vi "Write Report.vi"(8 "error in (no error)":errorcluster, 10 "Resource In":variant, 11 "Analyze Compound Results Base in":refnum<class "Analyze Compound Results Base.lvclass">) -> (0 "error out":errorcluster, 2 "Resource Out":variant, 3 "Analyze Compound Results Base out":refnum<class "Analyze Compound Results Base.lvclass">)   [LabVIEW 2014, in "Analyze Compound Results Base.lvclass"]
uses:
  Analyze Compound Results Base.lvclass
  Analyze Compound Results Base.lvclass/Analyze Compound Results Base.ctl
  Results Base/Analyze Results Base.lvclass
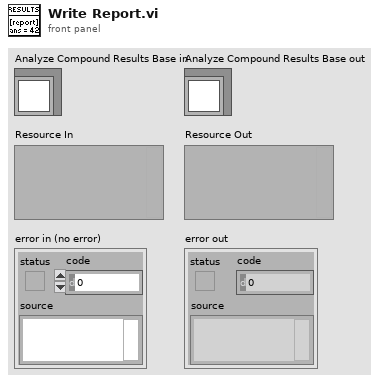
[diagram p1: front panel]
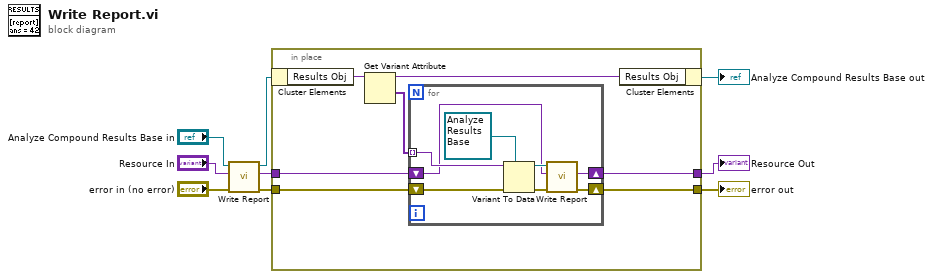
[diagram p0: block diagram]
diagram:
  n1 = call-parent "Write Report.vi"("error in (no error)"="error in (no error)", "Resource In"="Resource In", "Analyze Results Base in"="Analyze Compound Results Base in") -> ("error out"=w5:errorcluster, "Resource Out"=w2:variant, "Analyze Results Base out"=w6:refnum<class "Analyze Compound Results Base.lvclass">)  [unwired: 6 in]
  n2 = in-place {
    in-place-border: [w13] -> w4
    in-place-border: [w12] -> w3
    in-place-border: w5 -> [w11]
    in-place-border: w2 -> [w10]
    n3 = in-place-cluster #1(w6) -> ("Results Obj"=w16:variant)
    n4 = Get Variant Attribute(Variant=w16) -> (duplicate Variant=w15:variant, values=w14:variant[])  [unwired: 3 in, 2 out]
    n5 = for {
      tunnel: w14 -> [w24] mode=indexing
      shift-right: [w20] -> w12
      shift-left: w10 -> [w17]
      shift-right: [w18] -> w13
      shift-left: w11 -> [w22]
      n6 = Variant To Data(error in=w22, type=refnum<class "Analyze Results Base.lvclass"> refnum ("Analyze Results Base.lvclass"), Variant=w24) -> (data=w21:refnum<class "Analyze Results Base.lvclass">, error out=w19:errorcluster)
      n7 = call-dynamic "Write Report.vi"("error in (no error)"=w19, "Resource In"=w17, "Analyze Results Base in"=w21) -> ("error out"=w18:errorcluster, "Resource Out"=w20:variant)  [unwired: 6 in, 1 out]
    }
    n8 = in-place-cluster #1("Results Obj"=w15) -> (→"Analyze Compound Results Base out":refnum<class "Analyze Compound Results Base.lvclass">)
  }
  "error out" <- w4
  "Resource Out" <- w3
